vi "VESC TEST.vi"() -> ()   [LabVIEW 2019]
uses:
  <vilib>/rvi/Emulation/niFpgaGetClockAttributes.vi
  <vilib>/rvi/Emulation/niFpgaSctlEmulationGetInTimedLoop.vi
  <vilib>/rvi/Emulation/niFpgaEmulationReportErrorSimple.vi
  <vilib>/rvi/Emulation/niFpgaCriticalErrorInLSC.vi
panel:
  in  "stop":bool
  in  "ID":u32 format="%x"
  in  "Control Value":fxp<+/-,32,16>
  in  "Control Mode":T1(ring)
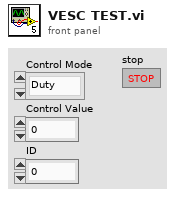
[diagram p1: front panel]
types:
  T1 = enum32{"Duty", "Current", "Brake", "RPM", "Position"}
  T2 = enum16{"100kBPS", "250kBPS", "500kBPS", "1000kBPS"}
  T3 = typedef "SPI Config.ctl" = cluster{"MXP Port":enum16{"A", "B"}, "Device":enum16{"CAN", "ENC", "IMU1", "IMU2"}, "CPOL":bool}
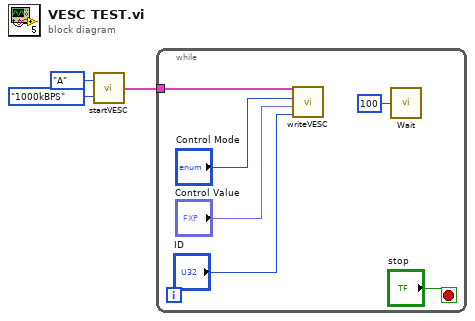
[diagram p0: block diagram]
diagram:
  n1 = call "startVESC.vi"("Baud Rate"=T2."1000kBPS", "MXP Port"=enum16{"A", "B"}."A") -> ("SPI Config Out"=w3:T3)
  n2 = while {
    tunnel: w3 -> [w9]
    stop <- "stop" stop-if-true
    n3 = call "writeVESC.vi"("ID"="ID", "Control Value"="Control Value", "Control Mode"="Control Mode", "SPI Config In"=w9) -> ()  [unwired: 1 out]
    n4 = call "Wait"("Count(mSec)"=u32 100) -> ()  [unwired: 1 out]
  }
